vi "CanAcceptDataDrag2.vi"(0 "XRef":T8, 1 "Point":T6, 2 "ProjectRef":T5, 3 "State In":T2) -> (14 "String?":T1, 15 "Path?":T1, 16 "Project Item?":T1)   [LabVIEW 2015, in "Async-And-Forget.xnode"]
doc: "This ability VI is used to specify whether your XNode can accept either string, path, or project item data drags. Currently Point is always (0, 0).\n\nDefault behavior: Reject data drags.\n\nThis ability does not provide UI and OS messages are not handled.\n\nSee also: OnDataDrag2, GetDataForDrag"
uses:
  Async-And-Forget.xnode
  <vilib>/XNodeSupport/XNodeXNodeRef.ctl
  <vilib>/XNodeSupport/XNodePoint.ctl
  <vilib>/XNodeSupport/XNodeInt.ctl
  <vilib>/XNodeSupport/XNodeProjectRef.ctl
  State.ctl
  <vilib>/Utility/miscctls.llb/LVRectTypeDef.ctl
  <vilib>/picture/picture.llb/imagedata.ctl
  <vilib>/XNodeSupport/XNodeBool.ctl
  <vilib>/XNodeSupport/NI_XNodeSupport.lvlib
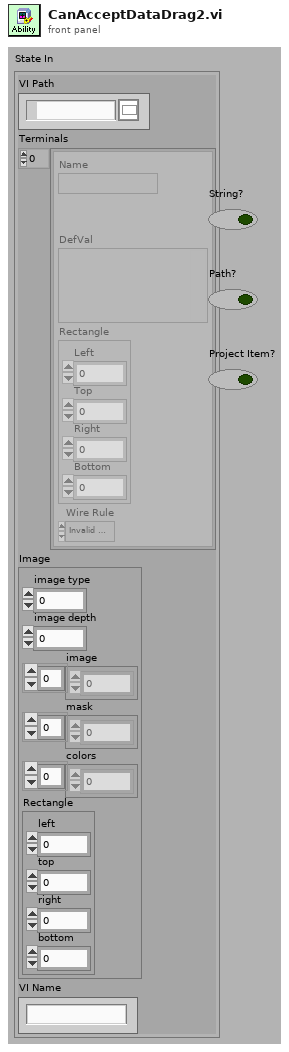
[diagram p1: front panel]
types:
  T1 = typedef "NI_XNodeSupport.lvlib/XNodeBool.ctl" = bool
  T2 = typedef "Async-And-Forget.xnode/State.ctl" = cluster{"VI Path":path, "Terminals":cluster{"Name":string, "DefVal":variant, "Rectangle":T3, "Wire Rule":enum16{"Invalid Wire Rule", "Required", "Recommended", "Optional", "Dynamic Dispatch"}}[], "Image":T4, "VI Name":string}
  T3 = typedef "LVRectTypeDef.ctl" = cluster{"Left":i16, "Top":i16, "Right":i16, "Bottom":i16}
  T4 = typedef "imagedata.ctl" = cluster{"image type":i32, "image depth":i32, "image":u8[], "mask":u8[], "colors":u32[], "Rectangle":cluster{"left":i16, "top":i16, "right":i16, "bottom":i16}}
  T5 = typedef "NI_XNodeSupport.lvlib/XNodeProjectRef.ctl" = refnum<vi>
  T6 = typedef "NI_XNodeSupport.lvlib/XNodePoint.ctl" = cluster{"H":T7, "V":T7}
  T7 = typedef "NI_XNodeSupport.lvlib/XNodeInt.ctl" = i32
  T8 = typedef "NI_XNodeSupport.lvlib/XNodeXNodeRef.ctl" = refnum<vi>
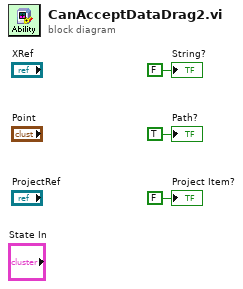
[diagram p0: block diagram]
diagram:
  "String?" <- T1 FALSE ("String?")
  "Path?" <- T1 TRUE ("Path?")
  "Project Item?" <- T1 FALSE ("Project Item?")
